vi "Start Sync.vi"(8 "error in (no error)":errorcluster, 10 "current time":timestamp, 11 "gRPC Server in":refnum<class "OCV4.lvclass">) -> (0 "error out":errorcluster, 3 "gRPC Server out":refnum<class "OCV4.lvclass">)   [LabVIEW 2019, in "OCV4.lvlib" / "OCV4.lvclass"]
uses:
  OCV4.lvclass
  OCV4.lvclass/OCV4.ctl
  RPC Messages/measurementservice_QueryResponse/measurementservice_QueryResponse_Data.ctl
  RPC Messages/measurementservice_ErrorOut/measurementservice_ErrorOut_Data.ctl
  RPC Messages/measurementservice_OCVRaw/measurementservice_OCVRaw_Data.ctl
  RPC Messages/measurementservice_OCVData/measurementservice_OCVData_Data.ctl
  RPC Messages/measurementservice_ACIRRaw/measurementservice_ACIRRaw_Data.ctl
  RPC Messages/measurementservice_ACIRData/measurementservice_ACIRData_Data.ctl
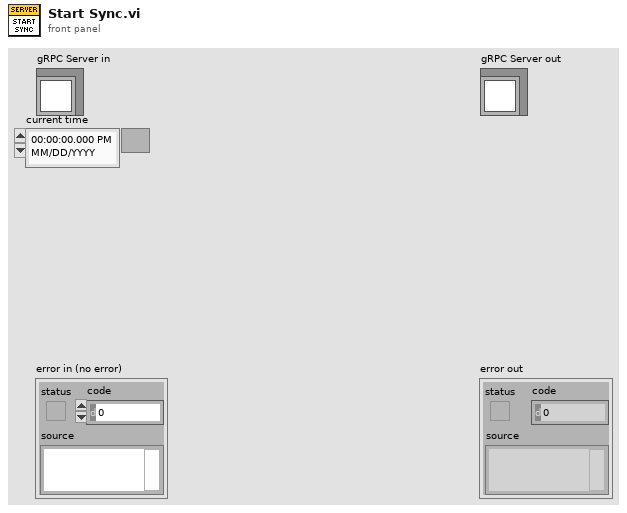
[diagram p1: front panel]
types:
  T1 = typedef "OCV4.lvlib/OCV4.lvclass/measurementservice_QueryResponse_Data.ctl" = cluster{"message":string, "status":i32}
  T2 = typedef "OCV4.lvlib/OCV4.lvclass/measurementservice_ErrorOut_Data.ctl" = cluster{"errCode":i32, "errMessage":string}
  T3 = typedef "OCV4.lvlib/OCV4.lvclass/measurementservice_OCVRaw_Data.ctl" = cluster{"battery1voltage":sgl, "battery2voltage":sgl, "battery3voltage":sgl, "error":T2}
  T4 = typedef "OCV4.lvlib/OCV4.lvclass/measurementservice_OCVData_Data.ctl" = cluster{"data":T3[]}
  T5 = typedef "OCV4.lvlib/OCV4.lvclass/measurementservice_ACIRRaw_Data.ctl" = cluster{"Impedance":sgl, "Real":sgl, "Imaginery":sgl, "error":T2}
  T6 = typedef "OCV4.lvlib/OCV4.lvclass/measurementservice_ACIRData_Data.ctl" = cluster{"data":T5[]}
  T7 = typedef "OCV4.lvlib/OCV4.lvclass/Server gRPC UEs.ctl" = cluster{"Invoke gRPC UE":refnum<user-event>, "Query gRPC UE":refnum<user-event>, "PerformOCVMeasurement gRPC UE":refnum<user-event>, "PerformACIRMeasurement gRPC UE":refnum<user-event>, "StreamOCVMeasurement gRPC UE":refnum<user-event>, "Register gRPC UE":refnum<user-event>}
  T8 = typedef "OCV4.lvlib/gprc-lvsupport.lvlib/grpcId.ctl" = u64
  T9 = typedef "OCV4.lvlib/OCV4.lvclass/measurementservice_QueryRequest_Data.ctl" = cluster{"query":string}
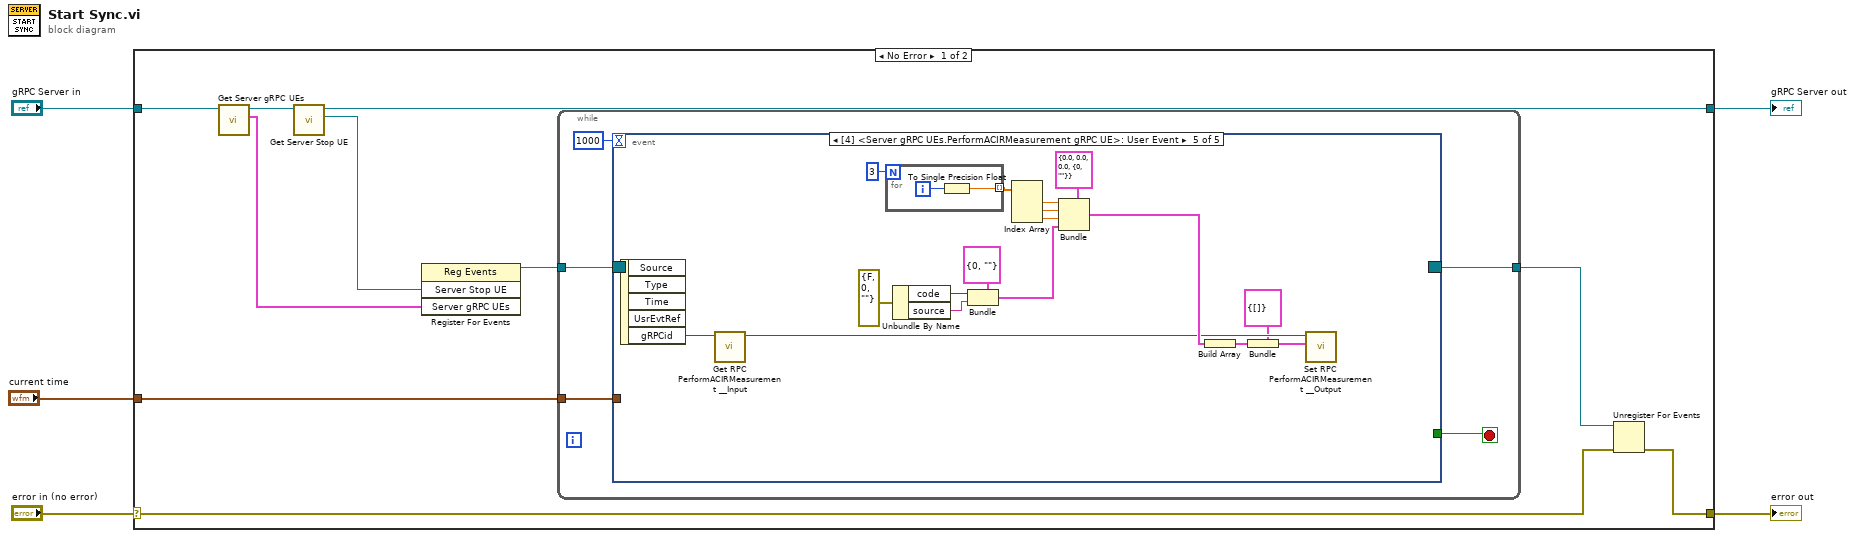
[diagram p0: block diagram]
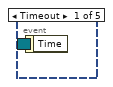
[diagram p2: hidden frame]
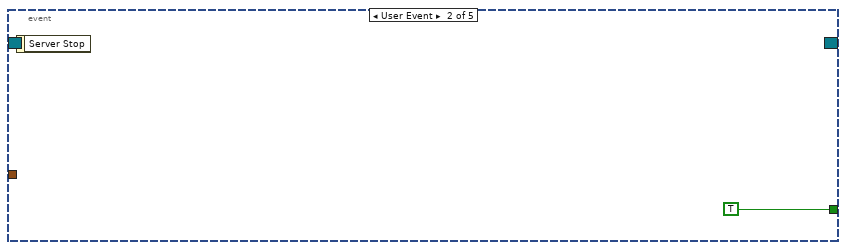
[diagram p3: hidden frame]
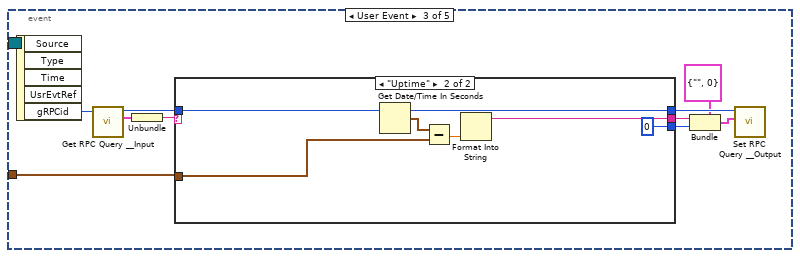
[diagram p4: hidden frame]
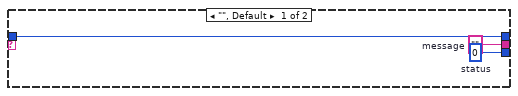
[diagram p5: hidden frame]
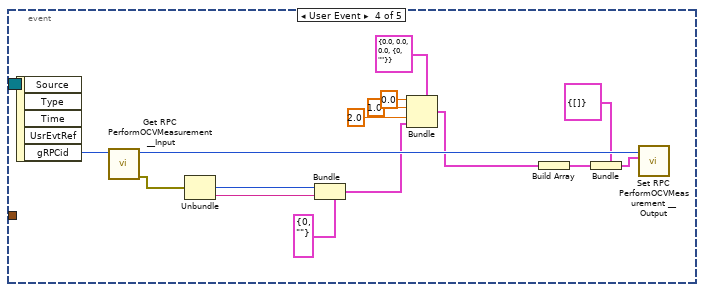
[diagram p6: hidden frame]
diagram:
  n1 = case shown="No Error" "error in (no error)" {
    selector: "error in (no error)" -> [w8 w76]
    tunnel: [w7 w76] -> w4
    tunnel: [w11 w75] -> w2
    tunnel: "gRPC Server in" -> [w15 w75]
    tunnel: "current time" -> [w6 _]
    frame No Error {
      n2 = call "Get Server gRPC UEs.vi"("OOP Server in"=w15) -> ("Server gRPC UEs"=w12:T7, "OOP Server out"=w14:refnum<class "OCV4.lvclass">)  [unwired: 9 in]
      n3 = call "Get Server Stop UE.vi"("OOP Server in"=w14) -> ("Server Stop UE"=w13:refnum<user-event>, "OOP Server out"=w11:refnum<class "OCV4.lvclass">)  [unwired: 9 in]
      n4 = register-events(w13, w12) -> (reference out=w10:refnum<event-registration>)  [unwired: 2 in, 1 out]
      n5 = while {
        tunnel: w10 -> [w20]
        tunnel: [w18] -> w9
        tunnel: w6 -> [w16]
        stop <- w19 stop-if-true
        n6 = event "RPC Methods Event Structure" shown="[4] <Server gRPC UEs.PerformACIRMeasurement gRPC UE>: User Event" {
          selector: w20 -> [_ _ _ _ _]
          dyn-events: [_ _ _ _ _] -> w18
          timeout: 1000 -> [_ _ _ _ _]
          tunnel: [_ TRUE _ _ _] -> w19
          tunnel: w16 -> [_ _ w22 _ _]
          event Timeout {
            n7 = event-data() -> ()  [unwired: 1 in, 1 out]
          }
          event User Event {
            n8 = event-data() -> ()  [unwired: 1 in, 1 out]
          }
          event User Event {
            n9 = event-data() -> ("gRPCid"=w23:T8)  [unwired: 1 in, 4 out]
            n10 = call "Get RPC Query __Input.vi"("gRPCid in"=w23) -> ("Message Data"=w30:T9, "gRPCid out"=w31:T8)  [unwired: 8 in, 1 out]
            n11 = Unbundle(w30) -> ("query"=w29:string)
            n12 = case shown="\"Uptime\"" w29 {
              tunnel: w31 -> [w34 w37]
              tunnel: [w34 w37] -> w28
              tunnel: [w33 w38] -> w26
              tunnel: [w32 0 ("status")] -> w25
              tunnel: w22 -> [_ w35]
              frame "", Default {
                w32 = 0  # status
                w33 = ""  # message
              }
              frame "Uptime" {
                n13 = Get Date/Time In Seconds() -> (seconds since 1Jan1904=w40:timestamp)
                n14 = Subtract(x=w40, y=w35) -> (x-y=w39:dbl)
                n15 = Format Into String(w39) -> (resulting string=w38:string)  [unwired: 3 in, 1 out]
              }
            }
            n16 = Bundle(cluster=T1 {"message"="", "status"=0} ("Message Data"), "message"=w26, "status"=w25) -> (w24:T1)
            n17 = call "Set RPC Query __Output.vi"("Message Data"=w24, "gRPCid in"=w28) -> ()  [unwired: 9 in, 1 out]
          }
          event User Event {
            n18 = event-data() -> ("gRPCid"=w41:T8)  [unwired: 1 in, 4 out]
            n19 = call "Get RPC PerformOCVMeasurement __Input.vi"("gRPCid in"=w41) -> ("error out"=w46:errorcluster, "gRPCid out"=w55:T8)  [unwired: 8 in, 1 out]
            n20 = Unbundle(w46) -> ("code"=w44:i32, "source"=w43:string)  [unwired: 1 out]
            n21 = Bundle(cluster=T2 {"errCode"=0, "errMessage"=""} ("measurementservice_ErrorOut_Data"), "errCode"=w44, "errMessage"=w43) -> (w42:T2)
            n22 = Bundle(cluster=T3 {"battery1voltage"=0.0, "battery2voltage"=0.0, "battery3voltage"=0.0, "error"={"errCode"=0, "errMessage"=""}} ("measurementservice_OCVRaw_Data"), "battery1voltage"=sgl 0.0, "battery2voltage"=sgl 1.0, "battery3voltage"=sgl 2.0, "error"=w42) -> (w51:T3)
            n23 = Build Array(w51) -> (w50:T3[])
            n24 = Bundle(cluster=T4 {"data"=[]} ("Message Data"), "data"=w50) -> (w53:T4)
            n25 = call "Set RPC PerformOCVMeasurement __Output.vi"("Message Data"=w53, "gRPCid in"=w55) -> ()  [unwired: 9 in, 1 out]
          }
          event User Event {
            n26 = event-data() -> ("gRPCid"=w56:T8)  [unwired: 1 in, 4 out]
            n27 = call "Get RPC PerformACIRMeasurement __Input.vi"("gRPCid in"=w56) -> ("gRPCid out"=w61:T8)  [unwired: 8 in, 2 out]
            n28 = for {
              N: 3 -> [_]
              tunnel: [w74] -> w65 mode=indexing
              i -> [w73]
              n29 = To Single Precision Float(number=w73) -> (single precision float=w74:sgl)
            }
            n30 = Unbundle By Name(errorcluster {"status"=FALSE, "code"=0, "source"=""} ("error in (no error)")) -> ("code"=w68:i32, "source"=w67:string)
            n31 = Bundle(cluster=T2 {"errCode"=0, "errMessage"=""} ("measurementservice_ErrorOut_Data"), "errCode"=w68, "errMessage"=w67) -> (w66:T2)
            n32 = Index Array(array=w65) -> (element #1=w64:sgl, element #2=w63:sgl, element #3=w62:sgl)  [unwired: 3 in]
            n33 = Bundle(cluster=T5 {"Impedance"=0.0, "Real"=0.0, "Imaginery"=0.0, "error"={"errCode"=0, "errMessage"=""}} ("measurementservice_ACIRRaw_Data"), "Impedance"=w64, "Real"=w63, "Imaginery"=w62, "error"=w66) -> (w69:T5)
            n34 = Build Array(w69) -> (w70:T5[])
            n35 = Bundle(cluster=T6 {"data"=[]} ("Message Data"), "data"=w70) -> (w59:T6)
            n36 = call "Set RPC PerformACIRMeasurement __Output.vi"("Message Data"=w59, "gRPCid in"=w61) -> ()  [unwired: 9 in, 1 out]
          }
        }
      }
      n37 = Unregister For Events(event registration refnum=w9, error in=w8) -> (error out=w7:errorcluster)
    }
    frame Error {
    }
  }
  "error out" <- w4
  "gRPC Server out" <- w2
